vi "Convert String to Boolean.vi"(11 "String":string) -> (2 "Valid string?":bool, 3 "Boolean value":bool)   [LabVIEW 2019, in "ProjectBuilder.lvlib"]
uses:
  ProjectBuilder.lvlib
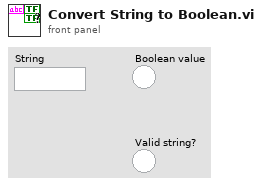
[diagram p1: front panel]
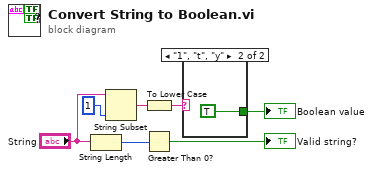
[diagram p0: block diagram]
diagram:
  n1 = String Length(string="String") -> (length=w6:i32)
  n2 = String Subset(string="String", length (rest)=1 ("length (rest)")) -> (substring=w2:string)  [unwired: 1 in]
  n3 = To Lower Case(string=w2) -> (all lower case string=w3:string)
  n4 = Greater Than 0?(x=w6) -> (x > 0?=→"Valid string?":bool)
  n5 = case shown="\"1\", \"t\", \"y\"" w3 {
    tunnel: [_ TRUE] -> w4
    frame Default {
    }
    frame "1", "t", "y" {
    }
  }
  "Boolean value" <- w4
